vi "32bit_to_8bit.vi"(8 "Numeric 6":u8, 9 "Numeric 5":u8, 10 "Numeric 4":u8, 11 "Numeric in":u8) -> (2 "Numeric out":dbl, 3 "Numeric 3":dbl)   [LabVIEW 2012]
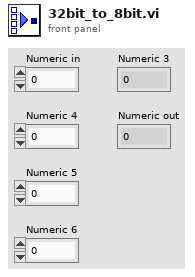
[diagram p1: front panel]
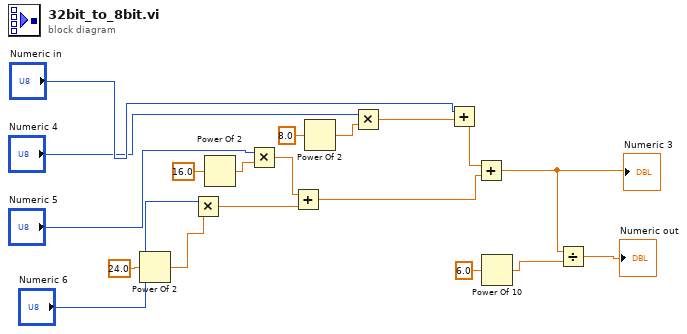
[diagram p0: block diagram]
diagram:
  n1 = Power Of 2(x=24.0) -> (2^x=w17:dbl)
  n2 = Multiply(x="Numeric 6", y=w17) -> (x*y=w18:dbl)
  n3 = Power Of 2(x=16.0) -> (2^x=w4:dbl)
  n4 = Multiply(x="Numeric 5", y=w4) -> (x*y=w9:dbl)
  n5 = Add(x=w9, y=w18) -> (x+y=w11:dbl)
  n6 = Power Of 2(x=8.0) -> (2^x=w8:dbl)
  n7 = Multiply(x="Numeric 4", y=w8) -> (x*y=w10:dbl)
  n8 = Add(x="Numeric in", y=w10) -> (x+y=w12:dbl)
  n9 = Add(x=w12, y=w11) -> (x+y=w13:dbl)
  "Numeric 3" <- w13
  n10 = Power Of 10(x=6.0) -> (10^x=w15:dbl)
  n11 = Divide(x=w13, y=w15) -> (x/y=→"Numeric out":dbl)
